vi "GPA.vi"() -> ()   [LabVIEW 2020]
panel:
  in  "?":bool
  in  "password":string
  in  "id":string
  in  "attendans":u8[](array[numeric]) max=10
  in  "bounas":u8[](array[numeric]) max=5
  out "Total GPA":dbl
  in  "Current GPA":dbl
  in  "Finished Units":dbl
  out "sum":dbl
  out "x*y":dbl[](array[numeric])
  out "GPA":dbl[](array[numeric])
  out "Total Units":u8
  out "Your GPA":dbl
  out "Subject State":string[](array[string])
  out "Final Indicator":bool[](array[boolean])
  out "Subject Grade":string[](array[string])
  out "Total Marks (100)":u8[](array[numeric])
  in  "Subject Units":u8[](array[numeric]) min=1 max=3
  in  "Subject Name":string[](array[string])
  in  "Final Marks (40)":u8[](array[numeric]) max=40
  in  "Mid-term Marks":u8[](array[numeric]) max=30
  in  "Quiz Marks (20)":u8[](array[numeric]) max=20
  # "GPA calculator Calculator For Maximum 8 Subjects"
  # "enter your id and password \n   your id            :2040794\n   your password: 0000\n enter 'login' to start calculation"
  # "your inputs for  semester"
  # "your results"
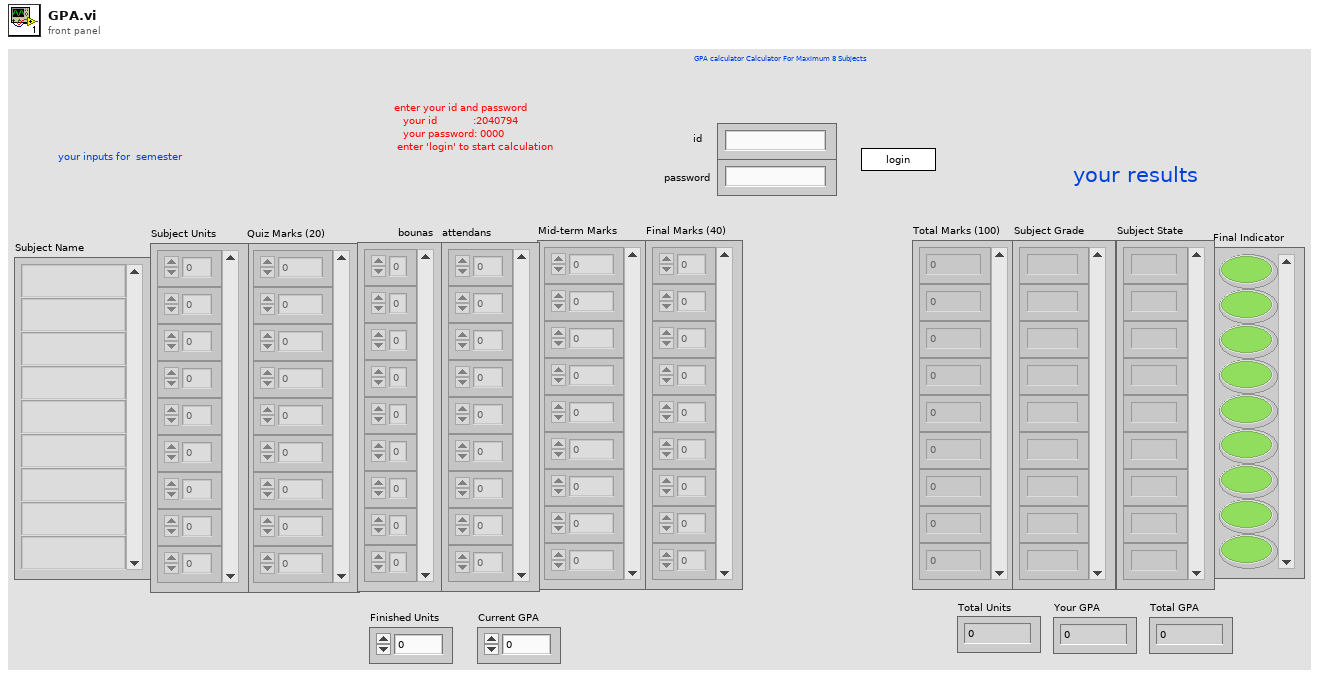
[diagram p1: front panel]
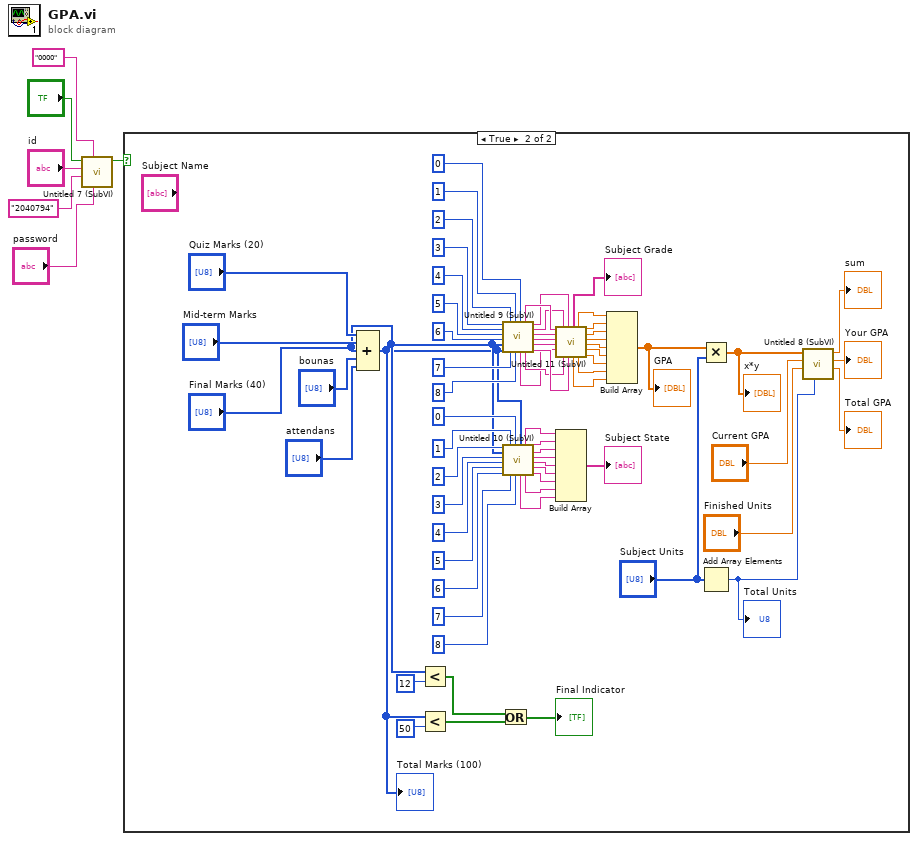
[diagram p0: block diagram]
diagram:
  n1 = call "Untitled 7 (SubVI).vi"("password"="password", "String"="0000", "String 2"="2040794", "id"="id", 11:"?") -> ("Boolean"=w1:bool)  [unwired: 6 in]
  n2 = case shown="True" w1 {
    frame False {
    }
    frame True {
      n3 = Compound Arithmetic op=ADD("Quiz Marks (20)", "Mid-term Marks", "Final Marks (40)", "bounas", "attendans") -> (w9:u8[])
      "Total Marks (100)" <- w9
      n4 = Less?(x="Final Marks (40)", y=12) -> (x < y?=w39:bool[])
      n5 = Less?(x=w9, y=50) -> (x < y?=w37:bool[])
      n6 = Or(x=w39, y=w37) -> (x .or. y?=→"Final Indicator":bool[])
      n7 = call "Untitled 9 (SubVI).vi"("index 6"=3 ("index"), "index"=4, "index 3"=5 ("index"), "index 4"=6 ("index"), "Final Marks (40)"="Final Marks (40)", "Array"=w9, "index 7"=2 ("index"), "index 5"=7 ("index"), "index 8"=1 ("index"), "index 2"=8, "index 9"=0 ("index")) -> ("String"=w23:string, "String 9"=w70:string, "String 2"=w60:string, "String 8"=w66:string, "String 7"=w65:string, "String 6"=w64:string, "String 5"=w63:string, "String 4"=w62:string, "String 3"=w61:string)
      n8 = call "Untitled 10 (SubVI).vi"("index 8"=2 ("index 2"), "Final Marks (40)"="Final Marks (40)", "index 7"=3 ("index 2"), "index 6"=4 ("index 2"), "index 5"=5 ("index 2"), "index 4"=6 ("index 2"), "index 9"=1 ("index 2"), "index 3"=7 ("index 2"), "index 10"=0 ("index 2"), "index in"=8 ("index 2"), "Array"=w9) -> ("s? t:f"=w21:string, "s? t:f 9"=w58:string, "s? t:f 2"=w44:string, "s? t:f 8"=w56:string, "s? t:f 7"=w49:string, "s? t:f 6"=w48:string, "s? t:f 5"=w47:string, "s? t:f 4"=w46:string, "s? t:f 3"=w45:string)
      n9 = call "Untitled 11 (SubVI).vi"("String 9"=w70, "String 6"=w64, "String 5"=w63, "String 4"=w62, "String"=w23, "String 7"=w65, "String 2"=w60, "String 8"=w66, "String 3"=w61) -> ("Array"=→"Subject Grade":string[], "s? t:f"=w18:dbl, "s? t:f 9"=w35:dbl, "s? t:f 2"=w28:dbl, "s? t:f 8"=w34:dbl, "s? t:f 7"=w33:dbl, "s? t:f 6"=w32:dbl, "s? t:f 5"=w31:dbl, "s? t:f 4"=w30:dbl, "s? t:f 3"=w29:dbl)  [unwired: 1 in]
      n10 = Build Array(w58, w56, w49, w48, w47, w46, w45, w44, w21) -> (→"Subject State":string[])
      n11 = Build Array(w35, w34, w33, w32, w31, w30, w29, w28, w18) -> (w26:dbl[])
      "GPA" <- w26
      n12 = Multiply(x=w26, y="Subject Units") -> (x*y=w25:dbl[])
      "x*y" <- w25
      n13 = Add Array Elements(numeric array="Subject Units") -> (sum=w14:u8)
      "Total Units" <- w14
      n14 = call "Untitled 8 (SubVI).vi"("Numeric Control"=w14, "Finished Units"="Finished Units", "Current GPA"="Current GPA", "Array"=w25) -> ("Numeric"=→"Total GPA":dbl, "Numeric 3"=→"Your GPA":dbl, "Numeric 2"=→"sum":dbl)  [unwired: 5 in]
    }
  }
